vi "Get Type.vi"(11 "Boolean in":refnum<class "Persistence.lvclass">) -> (3 "Type":string)   [LabVIEW 2017, in "Custom Type Test Executive.lvlib" / "Persistence.lvclass"]
uses:
  <vilib>/gpm_packages/@cs/test-executive/Source/Custom Type Test Executive/Persistence Data Type/Persistence.lvclass
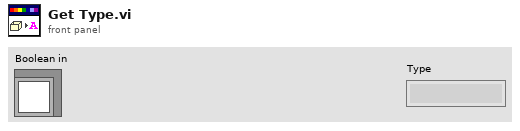
[diagram p1: front panel]
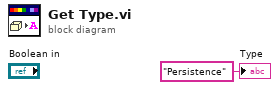
[diagram p0: block diagram]
diagram:
  "Type" <- "Persistence" ("Type")
